vi "Get Computer ID from NI Licence Manager.vi"(8 "error in (no error)":errorcluster, 11 "licence manager path":path) -> (0 "error out":errorcluster, 2 "computer name":string, 3 "computer ID":string)   [LabVIEW 2013]
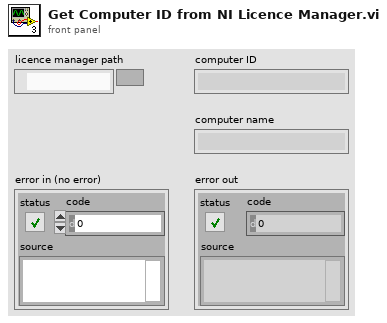
[diagram p1: front panel]
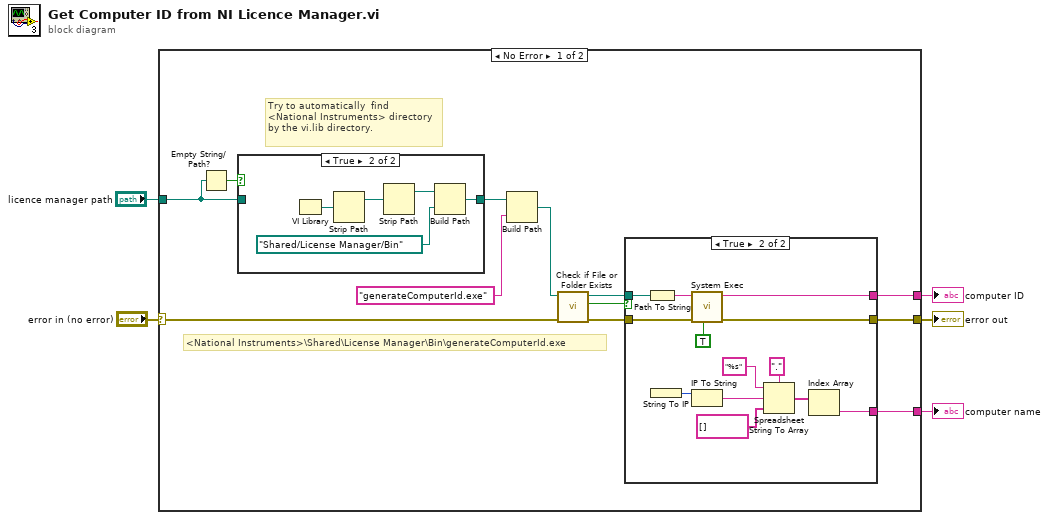
[diagram p0: block diagram]
diagram:
  n1 = case shown="No Error" "error in (no error)" {
    selector: "error in (no error)" -> [w6 w38]
    tunnel: "licence manager path" -> [w16 _]
    tunnel: [w9 _] -> w4
    tunnel: [w8 _] -> w3
    tunnel: [w7 w38] -> w2
    frame No Error {
      # "Try to automatically  find <National Instruments> directory by the vi.lib directory."
      # "<National Instruments>\\Shared\\License Manager\\Bin\\generateComputerId.exe"
      n2 = Empty String/Path?(string/path=w16) -> (empty?=w17:bool)
      n3 = case shown="True" w17 {
        tunnel: w16 -> [w32 _]
        tunnel: [w32 w33] -> w15
        frame False {
        }
        frame True {
          n4 = VI Library() -> (path=w37:path)
          n5 = Strip Path(path=w37) -> (stripped path=w36:path)  [unwired: 1 out]
          n6 = Strip Path(path=w36) -> (stripped path=w35:path)  [unwired: 1 out]
          n7 = Build Path(base path=w35, name or relative path=path "Shared/License Manager/Bin") -> (appended path=w33:path)
        }
      }
      n8 = Build Path(base path=w15, name or relative path="generateComputerId.exe" ("command line")) -> (appended path=w13:path)
      n9 = call <vilib>:"Check if File or Folder Exists.vi"("error in (no error)"=w6, "path"=w13) -> ("error out"=w11:errorcluster, "file or folder exists?"=w10:bool, "dup path"=w12:path)  [unwired: 7 in]
      n10 = case shown="True" w10 {
        tunnel: [_ w30] -> w8
        tunnel: [_ w19] -> w9
        tunnel: w12 -> [_ w27]
        tunnel: w11 -> [w18 w26]
        tunnel: [w18 w25] -> w7
        frame False {
        }
        frame True {
          n11 = Path To String(path=w27) -> (string=w28:string)
          n12 = String To IP() -> (0:w29:u32)  [unwired: 1 in]
          n13 = call <vilib>:"System Exec.vi"("run minimized? (F)"=TRUE, "error in (no error)"=w26, "command line"=w28) -> ("error out"=w25:errorcluster, "standard output"=w30:string)  [unwired: 5 in, 2 out]
          n14 = IP To String(2:w29) -> (0:w23:string)  [unwired: 1 in]
          n15 = Spreadsheet String To Array(delimiter (Tab)=".", format string="%s", spreadsheet string=w23, array type (2D Dbl)=string[] []) -> (array=w20:string[])
          n16 = Index Array(array=w20) -> (element=w19:string)  [unwired: 1 in]
        }
      }
    }
    frame Error {
    }
  }
  "computer name" <- w4
  "computer ID" <- w3
  "error out" <- w2
